vi "HiveMQ_Client.vi"(10 "Client Name":string="Client1", 11 "project namespace":string="LabVIEWDemo") -> ()   [LabVIEW 2017]
uses:
  <vilib>/LabVIEW Open Source Project/MQTT Broker/Control Packets/CONNACK/Connect Return Code -- enum.ctl
  <vilib>/LabVIEW Open Source Project/MQTT Broker/Client/Client.lvclass/Client.ctl
  e0c3b5cc-3527-4257-8471-923edf8b9748.vi
  <vilib>/LabVIEW Open Source Project/MQTT Broker/Client/Client.lvclass
  C:/Program Files (x86)/National Instruments/LabVIEW 2017/vi.lib/LabVIEW Open Source Project/MQTT Broker/MQTT_Base/MQTT_Base.lvclass
  <vilib>/LabVIEW Open Source Project/MQTT Broker/MQTT_Base/Decode Publish Package.vi
  <vilib>/LabVIEW Open Source Project/MQTT Broker/Control Packets/PUBLISH/PUBLISH.lvclass
  <vilib>/LabVIEW Open Source Project/MQTT Broker/MQTT_Base/MQTT_Base.lvclass
  <vilib>/LabVIEW Open Source Project/MQTT Broker/Control Packets/CONNACK/CONNACK.lvclass
panel:
  in  "period (ms)":i32=200
  in  "State History":i32(listbox)
  out "state":i32
  in  "subscribe":bool
  out "Topic":string
  out "Return Code":T1=enum."Server Unavailable"
  out "connected":bool
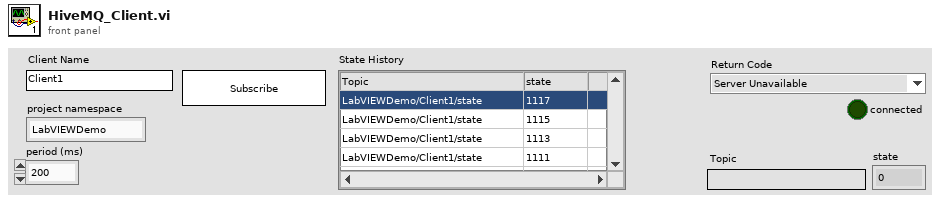
[diagram p1: front panel]
types:
  T1 = typedef "CONNACK.lvclass/Connect Return Code -- enum.ctl" = enum16{"Connection accepted", "Unacceptable protocol version", "Identifier Rejected", "Server Unavailable", "Bad Username or Password", "Not Authorized"}
  T2 = typedef "MQTT Server.lvlib/Client.lvclass/Public Events -- cluster.ctl" = cluster{"Connection Status":refnum<user-event>, "Connected":refnum<user-event>, "Application Message":refnum<user-event>}
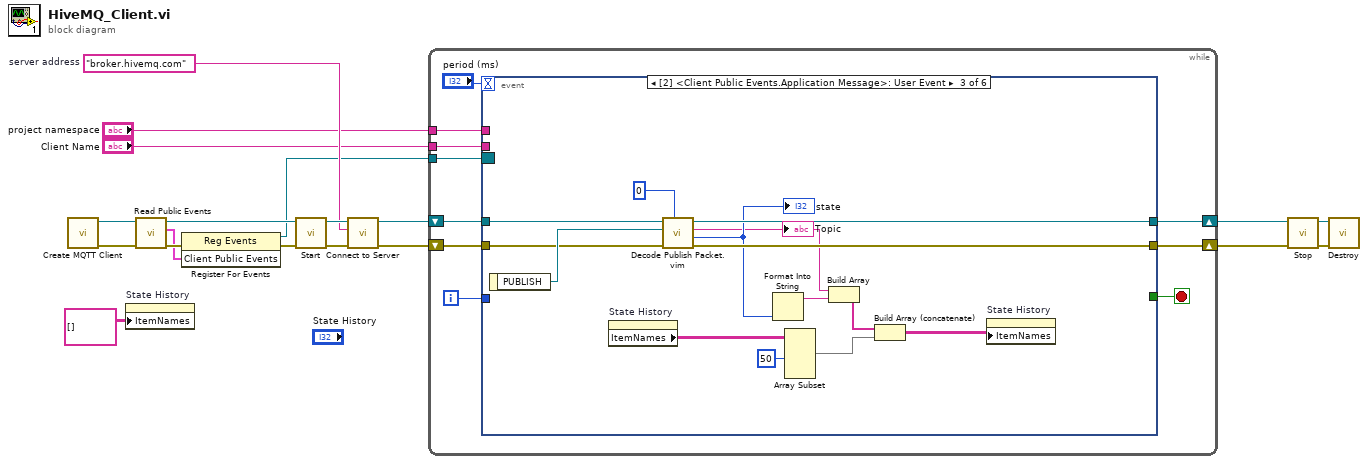
[diagram p0: block diagram]
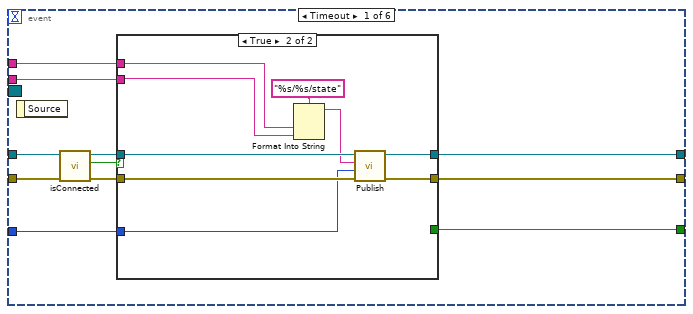
[diagram p2: hidden frame]
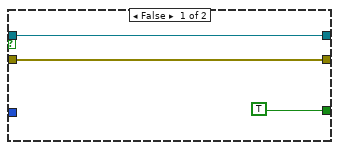
[diagram p3: hidden frame]
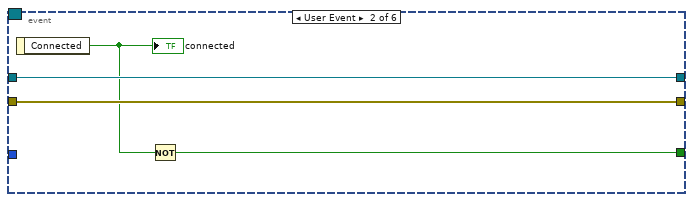
[diagram p4: hidden frame]
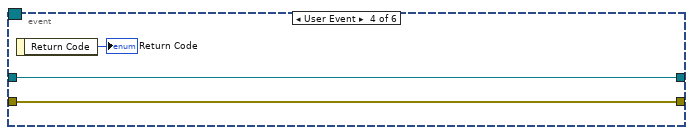
[diagram p5: hidden frame]
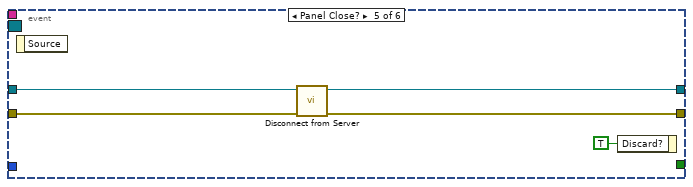
[diagram p6: hidden frame]
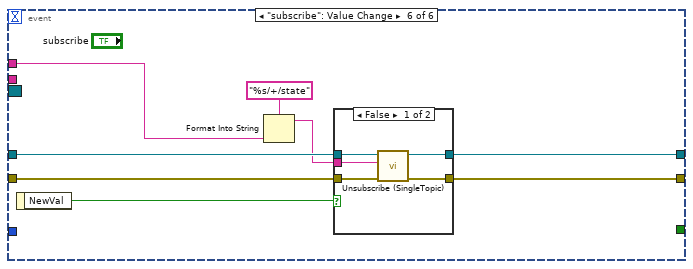
[diagram p7: hidden frame]
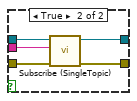
[diagram p8: hidden frame]
diagram:
  w16 = "broker.hivemq.com"  # server address
  n1 = call <vilib>:"Create MQTT Client.vi"() -> ("error out"=w15:errorcluster, "Client out"=w19:refnum<class "Client.lvclass">)  [unwired: 10 in]
  n2 = property on="State History" class="MCListbox (strict)"("ItemNames"=string[][] [] ("Item Names")) -> ()  [unwired: 2 in, 2 out]
  n3 = call <vilib>:"Read Public Events.vi"("error in (no error)"=w15, "Client in"=w19) -> ("error out"=w14:errorcluster, "Client Public Events"=w12:T2, "Client out"=w18:refnum<class "Client.lvclass">)  [unwired: 7 in]
  n4 = register-events(error in=w14, w12) -> (reference out=w9:refnum<event-registration>, error out=w13:errorcluster)  [unwired: 1 in]
  n5 = call <vilib>:"Start.vi"("error in (no error)"=w13, "MQTT_Base in"=w18) -> ("error out"=w11:errorcluster, "MQTT_Base out"=w17:refnum<class "Client.lvclass">)  [unwired: 7 in, 1 out]
  n6 = call <vilib>:"Connect to Server.vi"("error in (no error)"=w11, "address (localhost)"=w16, "Client in"=w17) -> ("error out"=w8:errorcluster, "Client out"=w10:refnum<class "Client.lvclass">)  [unwired: 5 in, 2 out]
  n7 = while {
    shift-right: [w25] -> w4
    shift-left: w10 -> [w28]
    tunnel: w9 -> [w27]
    shift-right: [w24] -> w3
    shift-left: w8 -> [w26]
    tunnel: "project namespace" -> [w22]
    tunnel: "Client Name" -> [w20]
    i -> [w21]
    stop <- w23 stop-if-true
    n8 = event shown="[2] <Client Public Events.Application Message>: User Event" {
      selector: w27 -> [_ _ _ _ _ _]
      dyn-events: _ -> [_ _ _ _ _ _]
      timeout: "period (ms)" -> [_ _ _ _ _ _]
      tunnel: w28 -> [w40 w56 w70 w72 w77 w86]
      tunnel: w26 -> [w39 w55 w67 w71 w75 w84]
      tunnel: [w37 w56 w69 w72 w76 w85] -> w25
      tunnel: [w35 w55 w66 w71 w74 w83] -> w24
      tunnel: [w31 w53 _ _ _ _] -> w23
      tunnel: w22 -> [w34 _ _ _ _ w82]
      tunnel: w21 -> [w33 _ _ _ _ _]
      tunnel: w20 -> [w30 _ _ _ _ _]
      event Timeout {
        n9 = event-data() -> ()  [unwired: 1 in, 1 out]
        n10 = call <vilib>:"isConnected.vi"("error in (no error)"=w39, "Client in"=w40) -> ("error out"=w36:errorcluster, "connected"=w32:bool, "Client out"=w38:refnum<class "Client.lvclass">)  [unwired: 7 in]
        n11 = case shown="True" w32 {
          tunnel: w38 -> [w43 w52]
          tunnel: [w43 w51] -> w37
          tunnel: w36 -> [w42 w50]
          tunnel: [w42 w49] -> w35
          tunnel: w34 -> [_ w47]
          tunnel: w33 -> [_ w45]
          tunnel: [TRUE _] -> w31
          tunnel: w30 -> [_ w44]
          frame False {
          }
          frame True {
            n12 = Format Into String(format string="%s/%s/state", w47, w44) -> (resulting string=w46:string)  [unwired: 2 in, 1 out]
            n13 = call <vilib>:"Publish.vi"("error in (no error)"=w50, "Payload"=w45, "Topic Name (empty: Payload name)"=w46, "Client in"=w52) -> ("error out"=w49:errorcluster, "Client out"=w51:refnum<class "Client.lvclass">)  [unwired: 5 in, 1 out]
          }
        }
      }
      event User Event {
        n14 = event-data() -> ("Connected"=w54:bool)  [unwired: 1 in]
        "connected" <- w54
        n15 = Not(x=w54) -> (.not. x?=w53:bool)
      }
      event User Event {
        n16 = event-data() -> ("PUBLISH"=w68:refnum<class "PUBLISH.lvclass">)  [unwired: 1 in]
        n17 = property on="State History" class="MCListbox (strict)"() -> ("ItemNames"=w59:string[][])  [unwired: 2 in, 2 out]
        n18 = call "Decode Publish Packet.vim"("Payload type"=0, "error in (no error)"=w67, "PUBLISH"=w68, "Client in"=w70) -> ("error out"=w66:errorcluster, "Payload"=w64:i32, "Topic"=w63:string, "Client out"=w69:refnum<class "Client.lvclass">)  [unwired: 4 in]
        "Topic" <- w63
        "state" <- w64
        n19 = Format Into String(w64) -> (resulting string=w62:string)  [unwired: 3 in, 1 out]
        n20 = Array Subset(array=w59, length (row)=50 ("length")) -> (w58:string[][])  [unwired: 3 in]
        n21 = Build Array(w63, w62) -> (w61:string[])
        n22 = Build Array (concatenate)(w61, w58) -> (w60:string[][])
        n23 = property on="State History" class="MCListbox (strict)"("ItemNames"=w60) -> ()  [unwired: 2 in, 2 out]
      }
      event User Event {
        n24 = event-data() -> ("Return Code"=→"Return Code":T1)  [unwired: 1 in]
      }
      event Panel Close? {
        n25 = event-data() -> ()  [unwired: 1 in, 1 out]
        n26 = call <vilib>:"Disconnect from Server.vi"("error in (no error)"=w75, "Client in"=w77) -> ("error out"=w74:errorcluster, "Client out"=w76:refnum<class "Client.lvclass">)  [unwired: 7 in, 1 out]
        n27 = event-data("Discard?"=TRUE) -> ()  [unwired: 1 in, 1 out]
      }
      event "subscribe": Value Change {
        n28 = event-data() -> ("NewVal"=w79:bool)  [unwired: 1 in]
        n29 = Format Into String(format string="%s/+/state", w82) -> (resulting string=w80:string)  [unwired: 2 in, 1 out]
        n30 = case shown="False" w79 {
          tunnel: w86 -> [w91 w96]
          tunnel: [w89 w95] -> w85
          tunnel: w84 -> [w88 w94]
          tunnel: [w87 w93] -> w83
          tunnel: w80 -> [w90 w92]
          frame False {
            n31 = call <vilib>:"Unsubscribe (SingleTopic).vi"("error in (no error)"=w88, "Topic Filter"=w90, "MQTT_Base in"=w91) -> ("error out"=w87:errorcluster, "MQTT_Base out"=w89:refnum<class "Client.lvclass">)  [unwired: 7 in]
          }
          frame True {
            n32 = call <vilib>:"Subscribe (SingleTopic).vi"("error in (no error)"=w94, "Topic Filter"=w92, "MQTT_Base in"=w96) -> ("error out"=w93:errorcluster, "MQTT_Base out"=w95:refnum<class "Client.lvclass">)  [unwired: 7 in]
          }
        }
      }
    }
  }
  n33 = call <vilib>:"Stop.vi"("error in (no error)"=w3, "MQTT_Base in"=w4) -> ("error out"=w6:errorcluster, "MQTT_Base out"=w7:refnum<class "Client.lvclass">)  [unwired: 7 in, 1 out]
  n34 = call-dynamic "Destroy.vi"("error in (no error)"=w6, "MQTT_Base in"=w7) -> ()  [unwired: 8 in, 2 out]
